vi "BusB Decode and Update.vi"(5 "In":u8[](array[numeric]), 7 "BusB TypeDef":T1, 11 "error in":errorcluster) -> (6 "BusB TypeDef out":T1, 15 "error out":errorcluster)   [LabVIEW 2016, in "Impedance Data Acquisition and Decoding.lvlib"]
uses:
  Impedance Data Acquisition and Decoding.lvlib
  <vilib>/imath/engines/lvmath2/RunTimeEngine/IndexRead/NIMS V(S).vi
  <vilib>/imath/engines/lvmath2/RunTimeEngine/ErrorHandling/NIMS_Create Error From Enums.vi
  <vilib>/imathl/engines/lvmath/Functions/Error Handling/Create Error.vi
  <vilib>/imath/engines/lvmath2/RunTimeEngine/NodeEndStatement/NIMS_NodeEndStatement_Output.vi
  <vilib>/imath/engines/lvmath2/RunTimeEngine/ErrorHandling/NIMS_Finalize Error.vi
  BusB Typedef.ctl
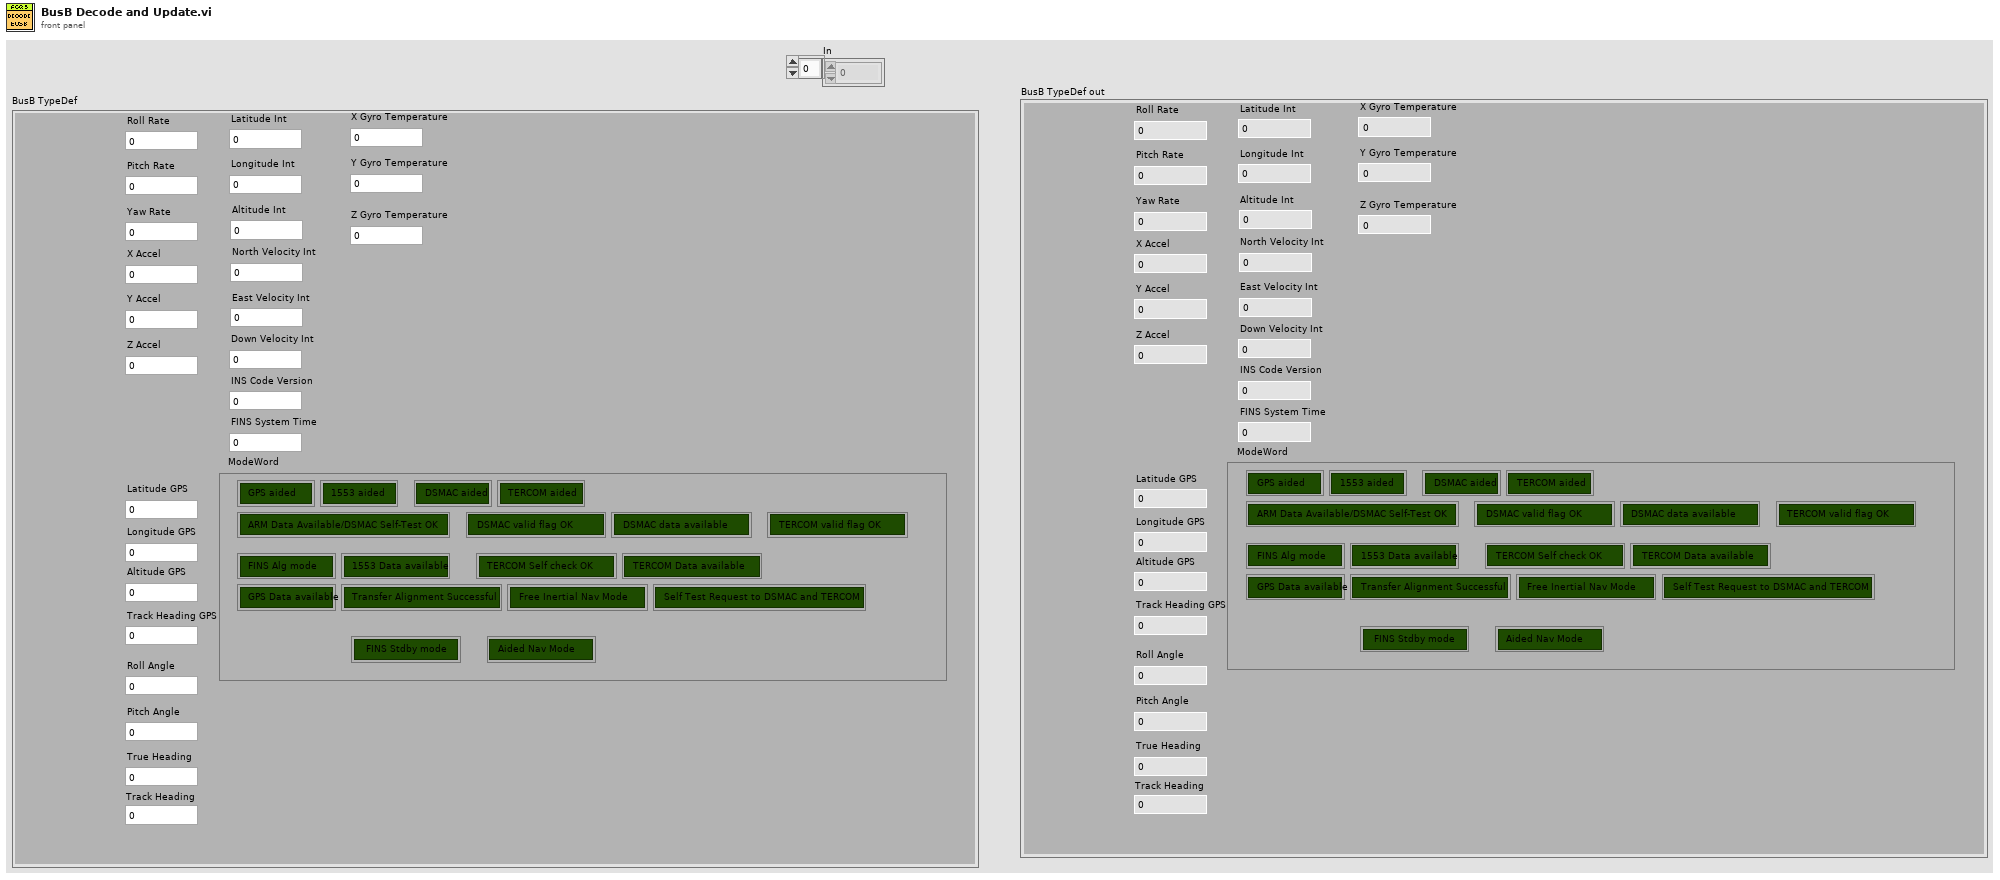
[diagram p1: front panel]
types:
  T1 = typedef "Impedance Data Acquisition and Decoding.lvlib/BusB Typedef.ctl" = cluster{"Pitch Rate":dbl, "Roll Rate":dbl, "Roll Angle":dbl, "Yaw Rate":dbl, "True Heading":dbl, "Pitch Angle":dbl, "Y Accel":dbl, "X Accel":dbl, "Z Accel":dbl, "X Gyro Temperature":dbl, "Longitude GPS":dbl, "Latitude GPS":dbl, "Altitude GPS":dbl, "Track Heading GPS":dbl, "Longitude Int":dbl, "Latitude Int":dbl, "Altitude Int":dbl, "FINS System Time":dbl, "East Velocity Int":dbl, "North Velocity Int":dbl, "INS Code Version":dbl, "ModeWord":cluster{"FINS Alg mode":bool, "GPS Data available":bool, "1553 Data available":bool, "Transfer Alignment Successful":bool, "TERCOM Self check OK":bool, "Free Inertial Nav Mode":bool, "TERCOM Data available":bool, "Self Test Request to DSMAC and TERCOM":bool, "ARM Data Available/DSMAC Self-Test OK":bool, "DSMAC valid flag OK":bool, "DSMAC data available":bool, "TERCOM valid flag OK":bool, "GPS aided":bool, "1553 aided":bool, "DSMAC aided":bool, "TERCOM aided":bool, "Aided Nav Mode":bool, " FINS Stdby mode":bool}, "Down Velocity Int":dbl, "Track Heading":dbl, "Y Gyro Temperature":dbl, "Z Gyro Temperature":dbl}
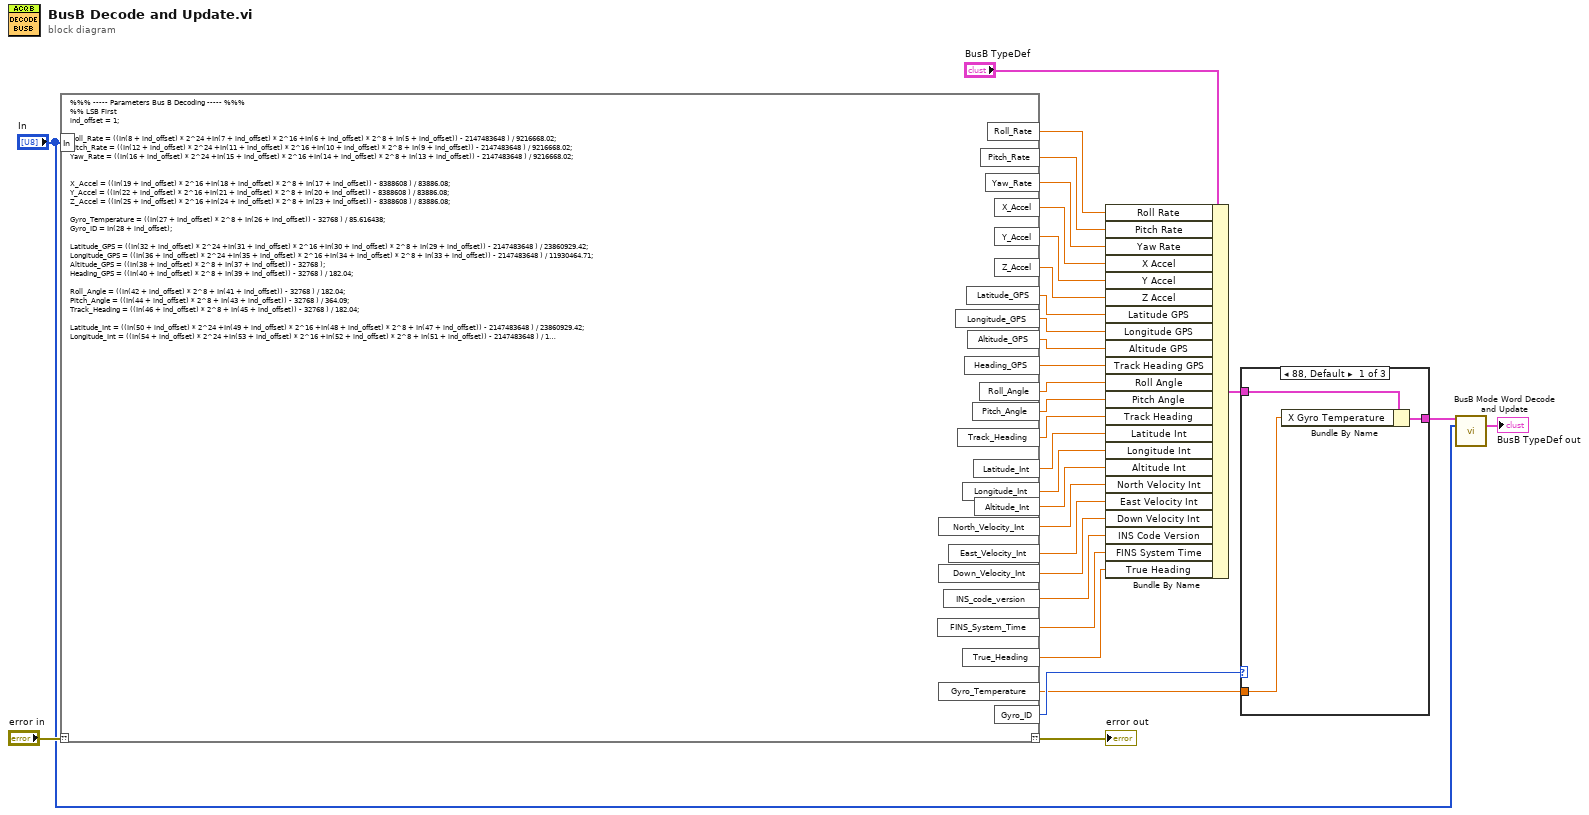
[diagram p0: block diagram]
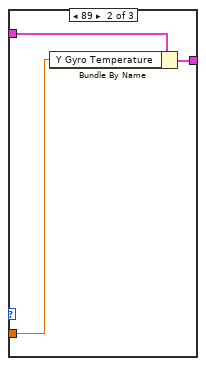
[diagram p2: hidden frame]
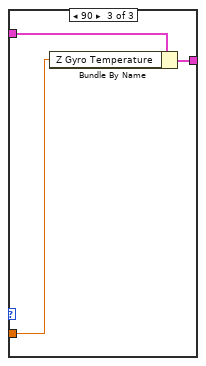
[diagram p3: hidden frame]
diagram:
  n1 = mathscript code="%%% ----- Parameters Bus B Decoding ----- %%%\n%% LSB First\nind_offset = 1;\n\nRoll_Rate = ((In(8 + ind_offset) * 2^24 +In(7 + ind_offset) * 2^16 +In(6 + ind_offset) * 2^8 + In(5 + ind_offset)) - 2147483648 ) / 9216668.02;\nPitch_Rate = ((In(12 + ind_offset) * 2^24 +In(11 + ind_offset) * 2^16 +In(10 + ind_offset) * 2^8 + In(9 + ind_offset)) - 2147483648 ) / 9216668.02;\nYaw_Rate = ((In(16 + ind_offset) * 2^24 +In(15 + ind_offset) * 2^16 +In(14 + ind_offset) * 2^8 + In(13 + ind_offset)) - 2147483648 ) / 9216668.02;\n\n\nX_Accel = ((In(19 + ind_offset) * 2^16 +In(18 + ind_offset) * 2^8 + In(17 + ind_offset)) - 8388608 ) / 83886.08;\nY_Accel = ((In(22 + ind_offset) * 2^16 +In(21 + ind_offset) * 2^8 + In(20 + ind_offset)) - 8388608 ) / 83886.08;\nZ_Accel = ((In(25 + ind_offset) * 2^16 +In(24 + ind_offset) * 2^8 + In(23 + ind_offset)) - 8388608 ) / 83886.08;\n\nGyro_Temperature = ((In(27 + ind_offset) * 2^8 + In(26 + ind_offset)) - 32768 ) / 85.616438;\nGyro_ID = In(28 + ind_offset);\n\nLatitude_GPS = ((In(32 + ind_offset) * 2^24 +In(31 + ind_offset) * 2^16 +In(30 + ind_offset) * 2^8 + In(29 + ind_offset)) - 2147483648 ) / 23860929.42;\nLongitude_GPS = ((In(36 + ind_offset) * 2^24 +In(35 + ind_offset) * 2^16 +In(34 + ind_offset) * 2^8 + In(33 + ind_offset)) - 2147483648 ) / 11930464.71;\nAltitude_GPS = ((In(38 + ind_offset) * 2^8 + In(37 + ind_offset)) - 32768 );\nHeading_GPS = ((In(40 + ind_offset) * 2^8 + In(39 + ind_offset)) - 32768 ) / 182.04;\n\nRoll_Angle = ((In(42 + ind_offset) * 2^8 + In(41 + ind_offset)) - 32768 ) / 182.04;\nPitch_Angle = ((In(44 + ind_offset) * 2^8 + In(43 + ind_offset)) - 32768 ) / 364.09;\nTrack_Heading = ((In(46 + ind_offset) * 2^8 + In(45 + ind_offset)) - 32768 ) / 182.04;\n\nLatitude_Int = ((In(50 + ind_offset) * 2^24 +In(49 + ind_offset) * 2^16 +In(48 + ind_offset) * 2^8 + In(47 + ind_offset)) - 2147483648 ) / 23860929.42;\nLongitude_Int = ((In(54 + ind_offset) * 2^24 +In(53 + ind_offset) * 2^16 +In(52 + ind_offset) * 2^8 + In(51 + ind_offset)) - 2147483648 ) / 11930464.71;\nAltitude_Int = ((In(56 + ind_offset) * 2^8 + In(55 + ind_offset)) - 32768 );\n\nNorth_Velocity_Int = ((In(58 + ind_offset) * 2^8 + In(57 + ind_offset)) - 32768 ) / 65.54;\nEast_Velocity_Int = ((In(60 + ind_offset) * 2^8 + In(59 + ind_offset)) - 32768 ) / 65.54;\nDown_Velocity_Int = ((In(62 + ind_offset) * 2^8 + In(61 + ind_offset)) - 32768 ) / 218.45;\n\n%% Skipping Modeword\n\nINS_code_version = In(65 + ind_offset)/100;\nTrue_Heading = ((In(67 + ind_offset) * 2^8 + In(66 + ind_offset)) - 32768 ) / 182.04;\n\nFINS_System_Time = (In(70 + ind_offset) * 2^16 +In(69 + ind_offset) * 2^8 + In(68 + ind_offset)) / 1000;"("??"="error in", "In"="In") -> ("??"=→"error out":errorcluster, "Roll_Rate"=w30:dbl, "Pitch_Rate"=w29:dbl, "Yaw_Rate"=w28:dbl, "X_Accel"=w27:dbl, "Y_Accel"=w26:dbl, "Z_Accel"=w25:dbl, "Gyro_Temperature"=w1:dbl, "Latitude_GPS"=w24:dbl, "Longitude_GPS"=w23:dbl, "Altitude_GPS"=w22:dbl, "Heading_GPS"=w21:dbl, "Roll_Angle"=w20:dbl, "Pitch_Angle"=w19:dbl, "Latitude_Int"=w18:dbl, "Longitude_Int"=w17:dbl, "Altitude_Int"=w16:dbl, "North_Velocity_Int"=w15:dbl, "East_Velocity_Int"=w14:dbl, "Down_Velocity_Int"=w13:dbl, "INS_code_version"=w12:dbl, "FINS_System_Time"=w11:dbl, "Track_Heading"=w10:dbl, "True_Heading"=w9:dbl, "Gyro_ID"=w2:u8)
  n2 = Bundle By Name(cluster="BusB TypeDef", "Roll Rate"=w30, "Pitch Rate"=w29, "Yaw Rate"=w28, "X Accel"=w27, "Y Accel"=w26, "Z Accel"=w25, "Latitude GPS"=w24, "Longitude GPS"=w23, "Altitude GPS"=w22, "Track Heading GPS"=w21, "Roll Angle"=w20, "Pitch Angle"=w19, "Track Heading"=w10, "Latitude Int"=w18, "Longitude Int"=w17, "Altitude Int"=w16, "North Velocity Int"=w15, "East Velocity Int"=w14, "Down Velocity Int"=w13, "INS Code Version"=w12, "FINS System Time"=w11, "True Heading"=w9) -> (w4:T1)
  n3 = case shown="88, Default" w2 {
    tunnel: w4 -> [w34 w37 w40]
    tunnel: [w33 w36 w39] -> w3
    tunnel: w1 -> [w32 w35 w38]
    frame 88, Default {
      n4 = Bundle By Name(cluster=w34, "X Gyro Temperature"=w32) -> (w33:T1)
    }
    frame 89 {
      n5 = Bundle By Name(cluster=w37, "Y Gyro Temperature"=w35) -> (w36:T1)
    }
    frame 90 {
      n6 = Bundle By Name(cluster=w40, "Z Gyro Temperature"=w38) -> (w39:T1)
    }
  }
  n7 = call "BusB Mode Word Decode and Update.vi"("BusB"=w3, "input bytes"="In") -> ("BusB out"=→"BusB TypeDef out":T1)  [unwired: 11 in, 2 out]
